vi "design buffer.vi"(8 "max buffer":i32=1000, 10 "action":enum16{"write", "read", "clear"}(ring), 11 "Design Inputs":T2) -> (0 "lost data":bool, 1 "got data":bool, 2 "buffer size":i32, 3 "Design Inputs Out":T2, 4 "more data":bool, 5 "User Project Design":T1[](array[typedef]), 6 "writes":i32, 7 "ADT Version":i32)   [LabVIEW 2015, in "AguaClara Library.lvlib"]
uses:
  AguaClara Library.lvlib
  user project design.ctl
  packed var.ctl
panel:
  out "reads":i32
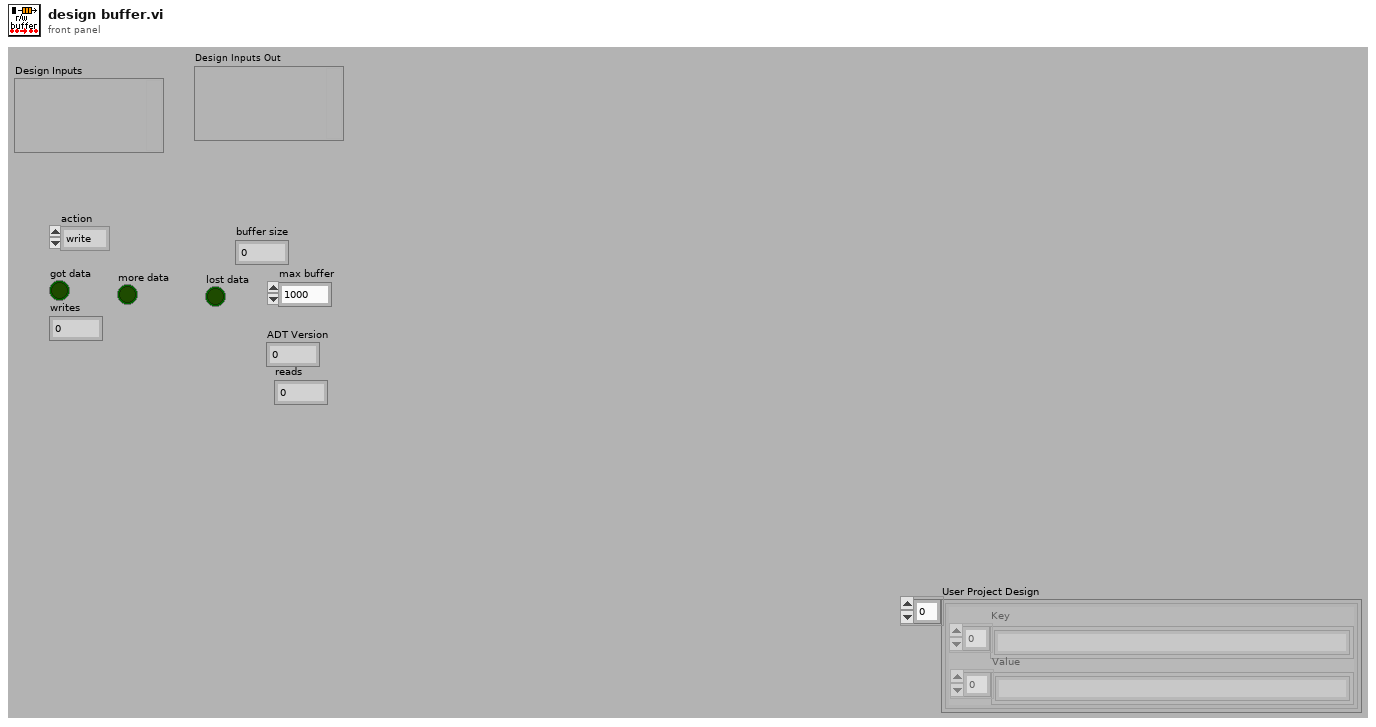
[diagram p1: front panel]
types:
  T1 = typedef "user project design.ctl" = cluster{"Key":string[], "Value":string[]}
  T2 = typedef "packed var.ctl" = variant
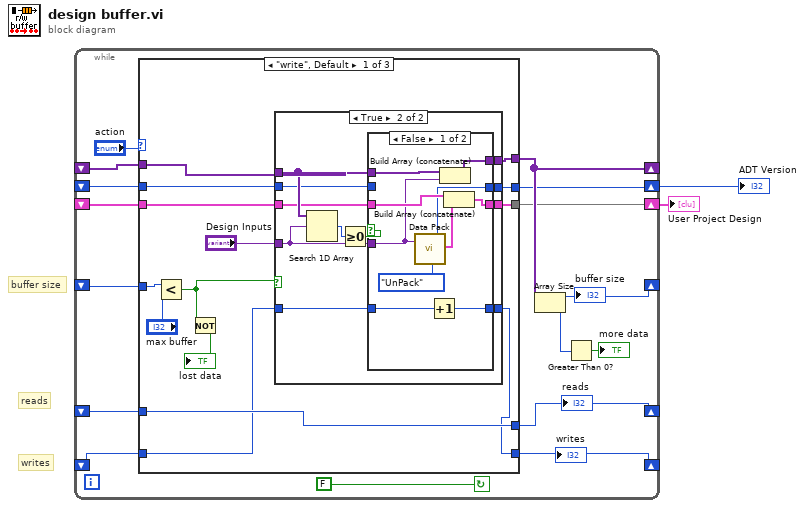
[diagram p0: block diagram]
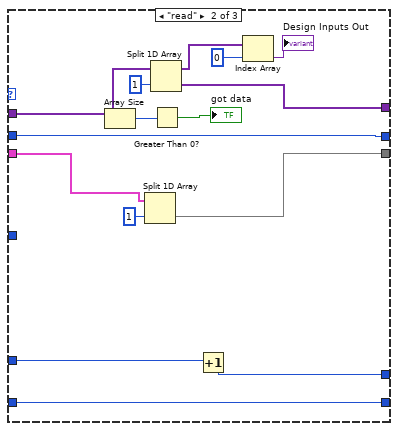
[diagram p4: hidden frame]
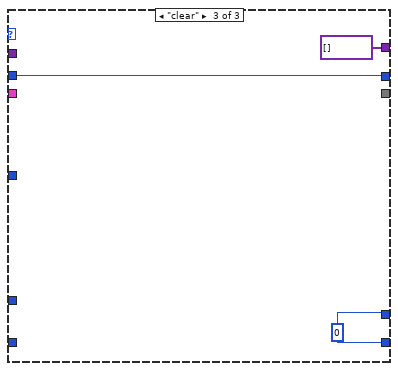
[diagram p5: hidden frame]
diagram:
  # "buffer size"
  # "writes"
  # "reads"
  n1 = while {
    shift-right: [w14] -> _
    shift-left: _ -> [w17]
    shift-right: [w12] -> _
    shift-left: _ -> [w13]
    shift-right: [w10] -> _
    shift-left: _ -> [w11]
    shift-right: [w9] -> _
    shift-left: _ -> [w7]
    shift-right: [w6] -> w2
    shift-left: _ -> [w5]
    shift-right: [w4] -> w1
    shift-left: _ -> [w3]
    stop <- FALSE continue-if-true
    n2 = case shown="\"write\", Default" "action" {
      tunnel: [w31 w74 variant[] []] -> w14
      tunnel: w17 -> [w29 w69 _]
      tunnel: w13 -> [w23 w68 _]
      tunnel: [w22 w68 w78] -> w12
      tunnel: [w30 w66 w78] -> w10
      tunnel: w11 -> [w30 w67 _]
      tunnel: w7 -> [w28 _ _]
      tunnel: [w21 w62 _] -> w6
      tunnel: w5 -> [w20 w63 _]
      tunnel: [w19 w61 w76] -> w4
      tunnel: w3 -> [w18 w61 w76]
      frame "write", Default {
        n3 = Less?(x=w28, y="max buffer") -> (x < y?=w25:bool)
        n4 = Not(x=w25) -> (.not. x?=→"lost data":bool)
        n5 = case shown="True" w25 {
          tunnel: [w35 w46] -> w31
          tunnel: w29 -> [w35 w45]
          tunnel: "Design Inputs" -> [_ w40]
          tunnel: w23 -> [w34 w42]
          tunnel: [w34 w41] -> w22
          tunnel: [w33 w39] -> w21
          tunnel: w20 -> [w33 w38]
          tunnel: [w32 w37] -> w19
          tunnel: w18 -> [w32 w36]
          frame False {
            # "buffer is full. Can't hold more in the queue"
          }
          frame True {
            n6 = Search 1D Array(1D array=w45, element=w40) -> (index of element=w44:i32)  [unwired: 1 in]
            n7 = Greater Or Equal To 0?(x=w44) -> (x >= 0?=w43:bool)
            n8 = case shown="False" w43 {
              tunnel: [w56 w60] -> w46
              tunnel: w40 -> [w50 _]
              tunnel: w45 -> [w55 w60]
              tunnel: w42 -> [w54 w59]
              tunnel: [w53 w59] -> w41
              tunnel: [w52 w58] -> w39
              tunnel: w38 -> [w51 w58]
              tunnel: [w48 w57] -> w37
              tunnel: w36 -> [_ w57]
              frame False {
                n9 = call "Data Pack.vi"("Packed In"=w50, "Data transform"=enum16{"Pack", "UnPack"}."UnPack") -> ("ADT version out"=w48:i32, "user project design"=w49:T1)  [unwired: 10 in, 6 out]
                n10 = Increment(x=w54) -> (x+1=w53:i32)
                n11 = Build Array (concatenate)(w55, w50) -> (w56:T2[])
                n12 = Build Array (concatenate)(w51, w49) -> (w52:T1[])
              }
              frame True {
              }
            }
          }
        }
      }
      frame "read" {
        n13 = Array Size(array=w69) -> (size(s)=w70:i32)
        n14 = Split 1D Array(array=w63, index=1) -> (second subarray=w62:T1[])  [unwired: 1 out]
        n15 = Split 1D Array(array=w69, index=1) -> (first subarray=w73:T2[], second subarray=w74:T2[])
        n16 = Greater Than 0?(x=w70) -> (x > 0?=→"got data":bool)
        n17 = Increment(x=w67) -> (x+1=w66:i32)
        n18 = Index Array(array=w73, index=0) -> (element=→"Design Inputs Out":T2)
      }
      frame "clear" {
        w78 = 0
      }
    }
    "writes" <- w12
    "reads" <- w10
    n19 = Array Size(array=w14) -> (size(s)=w9:i32)
    "buffer size" <- w9
    n20 = Greater Than 0?(x=w9) -> (x > 0?=→"more data":bool)
  }
  "User Project Design" <- w2
  "ADT Version" <- w1
